vi "Z6_Beamline.Calc State.vi"(0 "i ref in":refnum<vi>, 5 "error in (no error)":errorcluster) -> (14 "i ref out":refnum<vi>, 19 "error out":errorcluster)   [LabVIEW 2014, in "Z6_Beamline.lvlib"]
doc: "This VI contains all the VIs necesarry to calculate the state of all the subsystems and finally to derive the sum signal."
uses:
  Z6_Beamline.lvlib
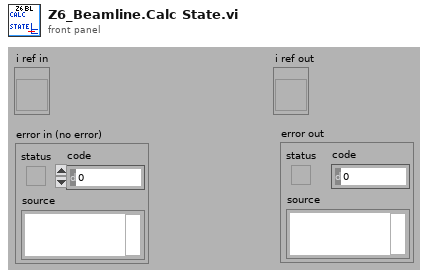
[diagram p1: front panel]
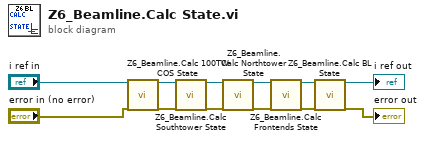
[diagram p0: block diagram]
diagram:
  n1 = call "Z6_Beamline.Calc 100TW COS State.vi"("i ref in"="i ref in", "error in (no error)"="error in (no error)") -> ("i ref out"=w3:refnum<vi>, "error out"=w5:errorcluster)  [unwired: 16 in]
  n2 = call "Z6_Beamline.Calc Southtower State.vi"("i ref in"=w3, "error in (no error)"=w5) -> ("i ref out"=w9:refnum<vi>, "error out"=w10:errorcluster)  [unwired: 16 in]
  n3 = call "Z6_Beamline.Calc Northtower State.vi"("i ref in"=w9, "error in (no error)"=w10) -> ("i ref out"=w6:refnum<vi>, "error out"=w7:errorcluster)  [unwired: 16 in]
  n4 = call "Z6_Beamline.Calc Frontends State.vi"("i ref in"=w6, "error in (no error)"=w7) -> ("i ref out"=w2:refnum<vi>, "error out"=w1:errorcluster)  [unwired: 16 in]
  n5 = call "Z6_Beamline.Calc BL State.vi"("i ref in"=w2, "error in (nop error)"=w1) -> ("i ref out"=→"i ref out":refnum<vi>, "error out"=→"error out":errorcluster)  [unwired: 16 in]
